vi "Write Template.vi"(8 "error in (no error)":errorcluster, 10 "Template":string, 11 "_Template in":refnum<class "_Template.lvclass">) -> (0 "error out":errorcluster, 3 "_Template out":refnum<class "_Template.lvclass">)   [LabVIEW 2021, in "_Template.lvlib" / "_Template.lvclass"]
uses:
  _Template.lvclass
  _Template.lvclass/_Template.ctl
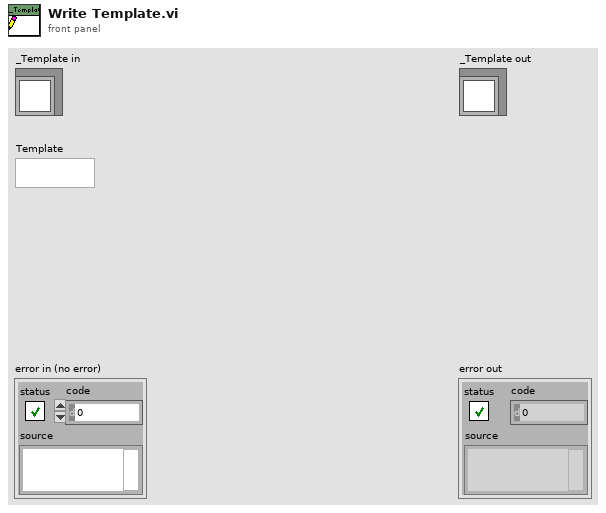
[diagram p1: front panel]
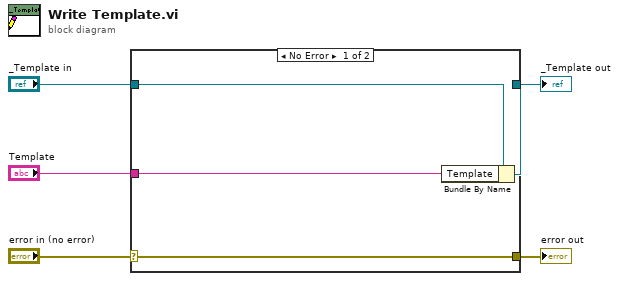
[diagram p0: block diagram]
diagram:
  n1 = case shown="No Error" "error in (no error)" {
    selector: "error in (no error)" -> [w9 w10]
    tunnel: [w9 w10] -> w4
    tunnel: [w7 w11] -> w2
    tunnel: "_Template in" -> [w8 w11]
    tunnel: "Template" -> [w6 _]
    frame No Error {
      n2 = Bundle By Name(cluster=w8, "Template"=w6) -> (w7:refnum<class "_Template.lvclass">)
    }
    frame Error {
    }
  }
  "error out" <- w4
  "_Template out" <- w2
